vi "Data to CSV.vi"(2 "Data Array":dbl[](array[numeric]), 3 "Precision (0)":i16, 4 "Units":string, 12 "String IN":string, 14 "Time? (F)":bool) -> (13 "String OUT":string)   [LabVIEW 2018]
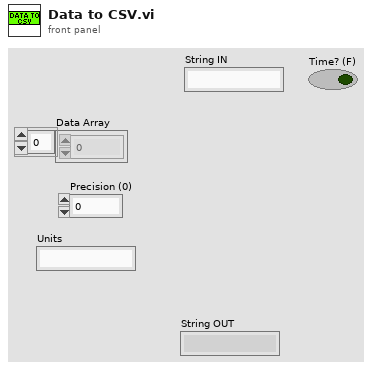
[diagram p1: front panel]
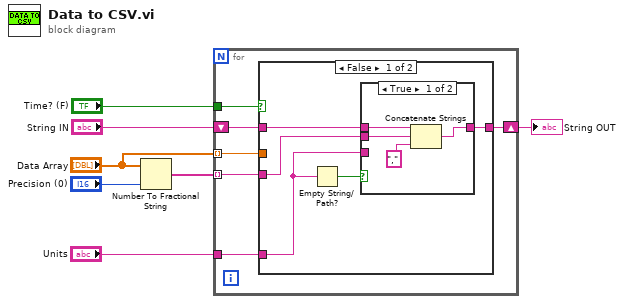
[diagram p0: block diagram]
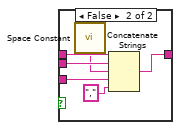
[diagram p2: hidden frame]
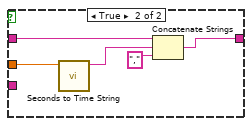
[diagram p3: hidden frame]
diagram:
  n1 = Number To Fractional String(number="Data Array", precision (6)="Precision (0)") -> (F-format string=w6:string[])  [unwired: 2 in]
  n2 = for {
    tunnel: w6 -> [w12] mode=indexing
    tunnel: "Units" -> [w11]
    shift-right: [w10] -> w3
    shift-left: "String IN" -> [w13]
    tunnel: "Time? (F)" -> [w9]
    tunnel: "Data Array" -> [w8] mode=indexing
    n3 = case shown="False" w9 {
      tunnel: w13 -> [w18 w33]
      tunnel: w12 -> [w17 _]
      tunnel: w11 -> [w14 _]
      tunnel: [w16 w32] -> w10
      tunnel: w8 -> [_ w30]
      frame False {
        n4 = Empty String/Path?(string/path=w14) -> (empty?=w15:bool)
        n5 = case shown="True" w15 {
          tunnel: w18 -> [w22 w28]
          tunnel: w17 -> [w21 w27]
          tunnel: w14 -> [_ w25]
          tunnel: [w20 w23] -> w16
          frame True {
            n6 = Concatenate Strings(w22, w21, "," ("string")) -> (w20:string)
          }
          frame False {
            n7 = call <vilib>:"Space Constant.vi"() -> ("String"=w26:string)
            n8 = Concatenate Strings(w28, w27, w26, w25, "," ("string")) -> (w23:string)
          }
        }
      }
      frame True {
        n9 = call "Seconds to Time String.vi"("Seconds"=w30) -> ("Time String"=w29:string)  [unwired: 10 in]
        n10 = Concatenate Strings(w33, w29, "," ("string")) -> (w32:string)
      }
    }
  }
  "String OUT" <- w3
